vi "1D B-Spline Fit.vi"(0 "Y":dbl[](array[numeric]), 1 "# of control points":i32=10, 5 "X":dbl[](array[numeric]), 7 "Weight":dbl[](array[numeric]), 12 "degree":i32=3, 13 "parameter selection":u16(ring)=2 items=["equally spaced", "chord length", "centripetal"]) -> (4 "Best BSpline Fit Y":dbl[](array[numeric]), 6 "Best BSpline Fit X":dbl[](array[numeric]), 14 "residue":dbl, 15 "error":i32)   [LabVIEW 2017, in "NI_AALPro.lvlib"]
doc: "Uses B-spline fitting to smooth a data set (<B>X</B>, <B>Y</B>)."
uses:
  NI_AALPro.lvlib
panel:
  # "1D B-Spline Fit"
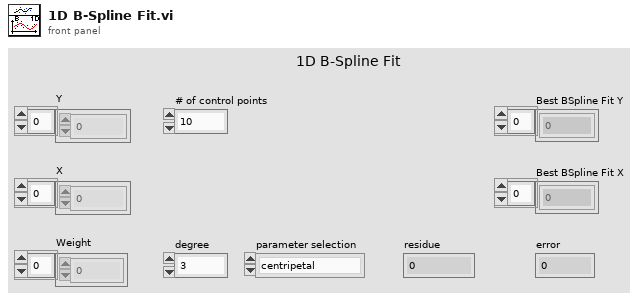
[diagram p1: front panel]
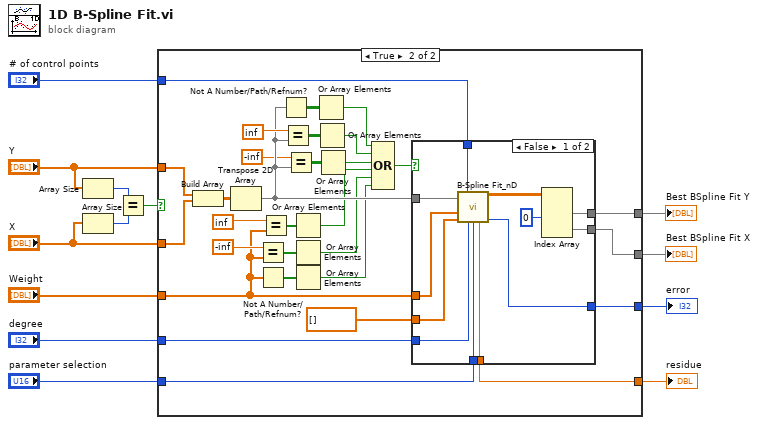
[diagram p0: block diagram]
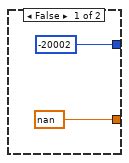
[diagram p2: hidden frame]
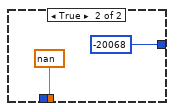
[diagram p3: hidden frame]
diagram:
  n1 = Array Size(array="Y") -> (size(s)=w6:i32)
  n2 = Array Size(array="X") -> (size(s)=w5:i32)
  n3 = Equal?(x=w6, y=w5) -> (x = y?=w4:bool)
  n4 = case shown="True" w4 {
    tunnel: "Y" -> [_ w45]
    tunnel: "X" -> [_ w44]
    tunnel: "# of control points" -> [_ w42]
    tunnel: "Weight" -> [_ w30]
    tunnel: "degree" -> [_ w41]
    tunnel: [_ w40] -> w11
    tunnel: [_ w39] -> w10
    tunnel: [nan ("residue") w38] -> w9
    tunnel: "parameter selection" -> [_ w37]
    tunnel: [-20002 ("error") w36] -> w7
    frame False {
    }
    frame True {
      n5 = Build Array(w45, w44) -> (w43:dbl[][])
      n6 = Transpose 2D Array(2D array=w43) -> (transposed array=w26:dbl[][])
      n7 = Equal?(x=-inf, y=w30) -> (x = y?=w28:bool[])
      n8 = Not A Number/Path/Refnum?(number/path/refnum=w30) -> (NaN/Path/Refnum?=w34:bool[])
      n9 = Equal?(x=inf, y=w30) -> (x = y?=w27:bool[])
      n10 = Not A Number/Path/Refnum?(number/path/refnum=w26) -> (NaN/Path/Refnum?=w35:bool[][])
      n11 = Equal?(x=inf, y=w26) -> (x = y?=w32:bool[][])
      n12 = Equal?(x=-inf, y=w26) -> (x = y?=w24:bool[][])
      n13 = Or Array Elements(Boolean array=w27) -> (logical OR=w19:bool)
      n14 = Or Array Elements(Boolean array=w28) -> (logical OR=w18:bool)
      n15 = Or Array Elements(Boolean array=w34) -> (logical OR=w17:bool)
      n16 = Or Array Elements(Boolean array=w35) -> (logical OR=w22:bool)
      n17 = Or Array Elements(Boolean array=w32) -> (logical OR=w21:bool)
      n18 = Or Array Elements(Boolean array=w24) -> (logical OR=w20:bool)
      n19 = Compound Arithmetic op=OR(w22, w21, w20, w19, w18, w17) -> (w16:bool)
      n20 = case shown="False" w16 {
        tunnel: w42 -> [w57 _]
        tunnel: w41 -> [w56 _]
        tunnel: [w53 _] -> w40
        tunnel: [w52 _] -> w39
        tunnel: [w51 nan ("residue")] -> w38
        tunnel: w37 -> [w50 _]
        tunnel: [w49 -20068 ("error")] -> w36
        tunnel: w30 -> [w48 _]
        tunnel: w26 -> [w47 _]
        tunnel: dbl[] [] ("parameter") -> [w46 _]
        frame False {
          n21 = call "B-Spline Fit_nD.vi"("Y"=w47, "# of control points"=w57, "Weight"=w48, "Parameter"=w46, "degree"=w56, "parameter selection"=w50) -> ("BSpline fit Y"=w55:dbl[][], "residue"=w51:dbl, "error"=w49:i32)  [unwired: 7 out]
          n22 = Index Array(array=w55, index (col) #1=0 ("disabled index (col)")) -> (element #1=w53:dbl[], element #2=w52:dbl[])  [unwired: 3 in]
        }
        frame True {
        }
      }
    }
  }
  "error" <- w7
  "Best BSpline Fit X" <- w10
  "residue" <- w9
  "Best BSpline Fit Y" <- w11
